vi "getstatus.vi"(8 "error in (no error)":errorcluster, 11 "MSCU":refnum<class "MSCU.lvclass">) -> (0 "error out":errorcluster, 2 "Status":string, 3 "MSCU":refnum<class "MSCU.lvclass">)   [LabVIEW 2019, in "MSCU.lvclass"]
uses:
  MSCU.lvclass
  MSCU.lvclass/MSCU.ctl
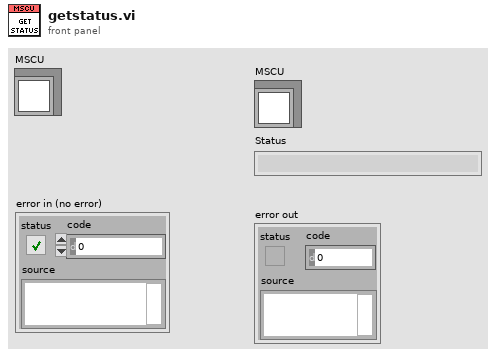
[diagram p1: front panel]
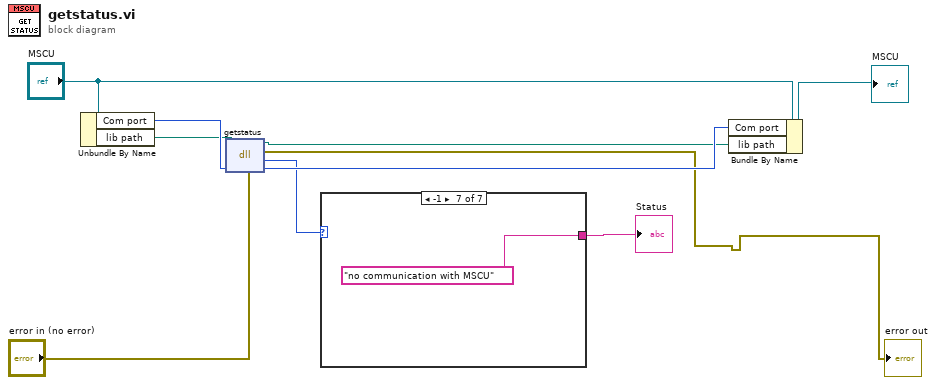
[diagram p0: block diagram]
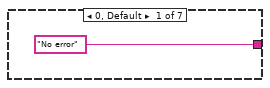
[diagram p2: hidden frame]
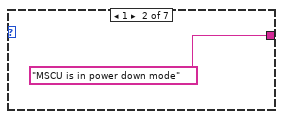
[diagram p3: hidden frame]
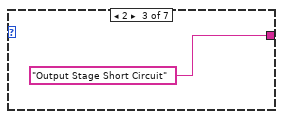
[diagram p4: hidden frame]
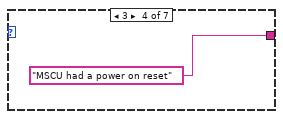
[diagram p5: hidden frame]
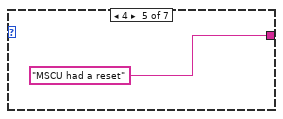
[diagram p6: hidden frame]
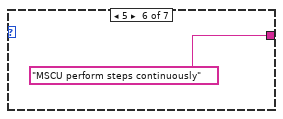
[diagram p7: hidden frame]
diagram:
  n1 = Unbundle By Name("MSCU") -> ("Com port"=w7:i32, "lib path"=w6:path)
  n2 = dll-call lib="C:/Program Files (x86)/Nanonis/SPM Controller/data/MSCU.dll" fn="getstatus"(path in=w6, error in="error in (no error)", "Comport"=w7) -> (path out=w4:path, error out=→"error out":errorcluster, "return type"=w8:i32, "Comport"=w10:i32)  [unwired: 1 in]
  n3 = case shown="-1" w8 {
    tunnel: ["No error" "MSCU is in power down mode" "Output Stage Short Circuit" "MSCU had a power on reset" "MSCU had a reset" "MSCU perform steps continuously" "no communication with MSCU"] -> w9
    frame 0, Default {
    }
    frame 1 {
    }
    frame 2 {
    }
    frame 3 {
    }
    frame 4 {
    }
    frame 5 {
    }
    frame -1 {
    }
  }
  "Status" <- w9
  n4 = Bundle By Name(cluster="MSCU", "Com port"=w10, "lib path"=w4) -> (→"MSCU":refnum<class "MSCU.lvclass">)
